vi "reserve or unreserve tree entry.vi"(8 "error in (no error)":errorcluster, 9 "Item Ref in":T1 format="%.0x", 10 "Tag":string, 11 "TreeControl in":refnum<vi>) -> (0 "error out":errorcluster)   [LabVIEW 2016, in "FPGA Addon System Explorer.lvlib"]
uses:
  FPGA Addon System Explorer.lvlib
  <vilib>/NI Veristand/Custom Device API/Custom Device Item Ref.ctl
  reservation type.ctl
  RM Client API/FPGA RM Client API.lvlib
  <vilib>/NI VeriStand/Custom Device API/Custom Device API.lvlib
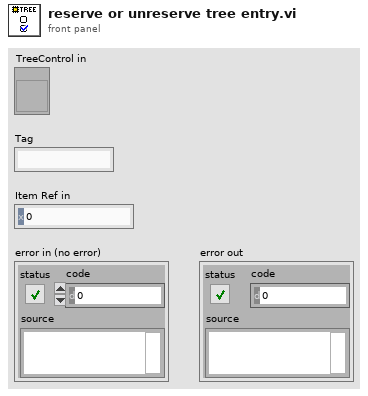
[diagram p1: front panel]
types:
  T1 = typedef "Custom Device API.lvlib/Custom Device Item Ref.ctl" = u64
  T2 = typedef "FPGA Addon System Explorer.lvlib/reservation type.ctl" = enum16{"none", "available", "reserved by this", "reserved by other", "incompatible", "parent"}
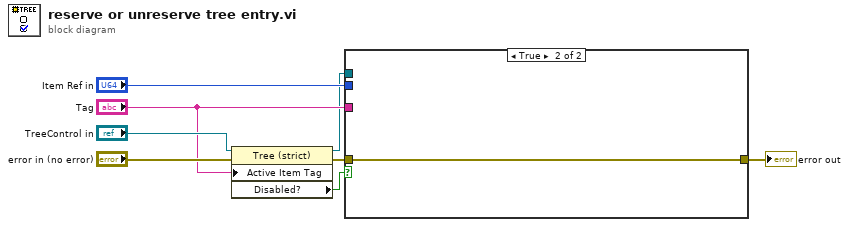
[diagram p0: block diagram]
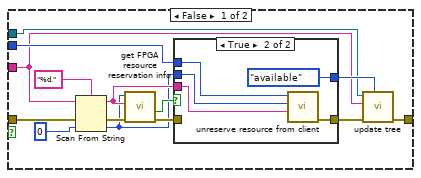
[diagram p2: hidden frame]
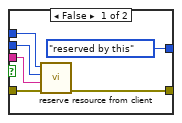
[diagram p3: hidden frame]
diagram:
  n1 = property class="Tree (strict)"(reference="TreeControl in", error in="error in (no error)", "Active Item Tag"="Tag") -> (reference out=w1:refnum<vi>, error out=w4:errorcluster, "Disabled?"=w3:bool)
  n2 = case shown="True" w3 {
    tunnel: [w21 w34] -> w8
    tunnel: w4 -> [w20 w34]
    tunnel: "Item Ref in" -> [w14 _]
    tunnel: "Tag" -> [w13 _]
    tunnel: w1 -> [w9 _]
    frame False {
      n3 = Scan From String(format string="%d.", input string=w13, error in=w20, default 1=u64 0 ("default value 1")) -> (remaining string=w16:string, error out=w19:errorcluster, output 1=w15:u64)  [unwired: 1 in, 1 out]
      n4 = call "get FPGA resource reservation info.vi"("error in (no error)"=w19, "Name in Bitfile"=w16, "Item Ref in"=w15) -> ("error out"=w18:errorcluster, "found?"=w17:bool)  [unwired: 4 in, 3 out]
      n5 = case shown="True" w17 {
        tunnel: [w24 w33] -> w12
        tunnel: w14 -> [w27 w32]
        tunnel: w15 -> [w28 w31]
        tunnel: w16 -> [w26 w30]
        tunnel: w18 -> [w25 _]
        tunnel: [reservation_type."reserved by this" ("status type") reservation_type."available" ("status type")] -> w22
        frame False {
          n6 = call "reserve resource from client.vi"("error in (no error)"=w25, "Name in Bitfile"=w26, "Server Ref in"=w28, "Item Ref in"=w27) -> ("error out"=w24:errorcluster)  [unwired: 6 in, 1 out]
        }
        frame True {
          n7 = call "unreserve resource from client.vi"("Name in Bitfile"=w30, "Server Ref in"=w31, "Item Ref in"=w32) -> ("error out"=w33:errorcluster)  [unwired: 7 in, 1 out]
        }
      }
      n8 = call "update tree.vi"("status type"=w22, "error in (no error)"=w12, "tag"=w13, "TreeControl in"=w9) -> ("error out"=w21:errorcluster)  [unwired: 7 in]
    }
    frame True {
    }
  }
  "error out" <- w8
